vi "Move All Objects on Diagram.vi"(6 "Delta Position":T1, 8 "error in (no error)":errorcluster, 11 "Diag Refnum":refnum<vi>) -> (0 "error out":errorcluster, 3 "Diag Refnum Out":refnum<vi>)   [LabVIEW 2012, in "Scripting Tools.lvlib"]
uses:
  Scripting Tools.lvlib
  <vilib>/Utility/miscctls.llb/LVBoundsTypeDef.ctl
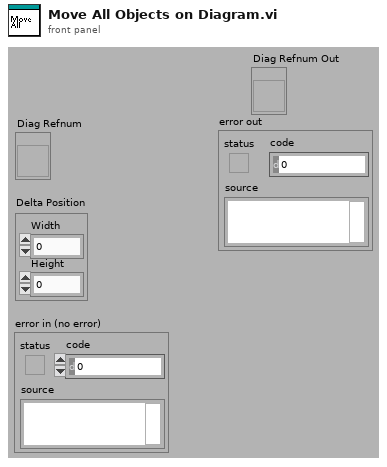
[diagram p1: front panel]
types:
  T1 = typedef "LVBoundsTypeDef.ctl" = cluster{"Width":u32, "Height":u32}
  T2 = typedef "LVPositionTypeDef.ctl" = cluster{"Left":i32, "Top":i32}
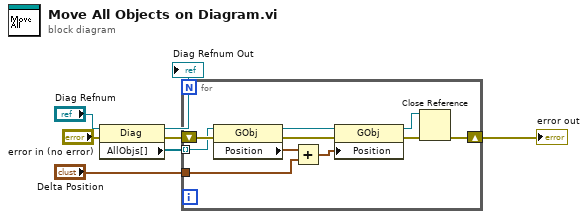
[diagram p0: block diagram]
diagram:
  n1 = property class="Diag"(reference="Diag Refnum", error in="error in (no error)") -> (reference out=→"Diag Refnum Out":refnum<vi>, error out=w4:errorcluster, "AllObjs[]"=w5:refnum<vi>[])
  n2 = for {
    shift-right: [w8] -> w1
    shift-left: w4 -> [w17]
    tunnel: w5 -> [w16] mode=indexing
    tunnel: "Delta Position" -> [w14]
    n3 = property class="GObj"(reference=w16, error in=w17) -> (reference out=w12:refnum<vi>, error out=w13:errorcluster, "Position"=w15:T2)
    n4 = Add(x=w15, y=w14) -> (x+y=w11:T1)
    n5 = property class="GObj"(reference=w12, error in=w13, "Position"=w11) -> (reference out=w9:refnum<vi>, error out=w10:errorcluster)
    n6 = Close Reference(reference=w9, error in (no error)=w10) -> (error out=w8:errorcluster)
  }
  "error out" <- w1
